vi "lua_pop.vi"(8 "error in (no error)":errorcluster, 10 "n":i32, 11 "lua_state_p":u64) -> (0 "error out":errorcluster, 3 "lua_state_p out":u64)   [LabVIEW 2020, in "lua.dll.lvlib"]
uses:
  lua.dll.lvlib
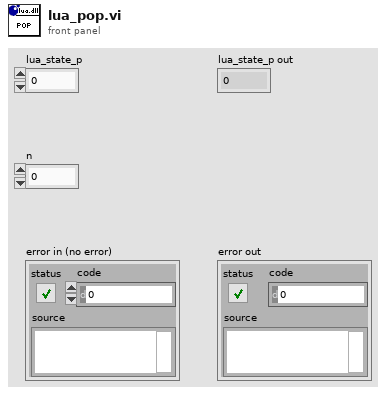
[diagram p1: front panel]
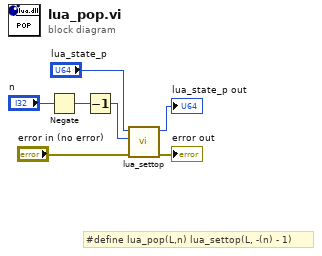
[diagram p0: block diagram]
diagram:
  # "#define lua_pop(L,n) lua_settop(L, -(n) - 1)"
  n1 = Negate(x="n") -> (-x=w6:i32)
  n2 = Decrement(x=w6) -> (x-1=w1:i32)
  n3 = call "lua_settop.vi"("error in (no error)"="error in (no error)", "index"=w1, "lua_state_p"="lua_state_p") -> ("error out"=→"error out":errorcluster, "lua_state_p out"=→"lua_state_p out":u64)  [unwired: 7 in]
